vi "getSpeedAndGainSettings.vi"(6 "Delay between send and receive [ms]":i32=100, 8 "error in (no error)":errorcluster, 11 "CCD in":refnum<class "CCD.lvclass">) -> (0 "error out":errorcluster, 1 "CCD-gain options":string[](array[string]), 2 "CCD-speed options":string[](array[string]), 3 "CCD out":refnum<class "CCD.lvclass">)   [LabVIEW 2023, in "CCD.lvclass"]
doc: "Wrapper around the getSpeed and getGain VIs for convenience."
uses:
  CCD.lvclass
  CCD.lvclass/CCD.ctl
  20f7d3bd-08ac-4524-9bed-df36c1da25a0.vi
  GenericDevice/GenericDevice.lvclass
  <vilib>/JDP Science/JSONtext/JSONtext.lvlib
panel:
  out "results-JSON string":string
  # "Connector Pane"
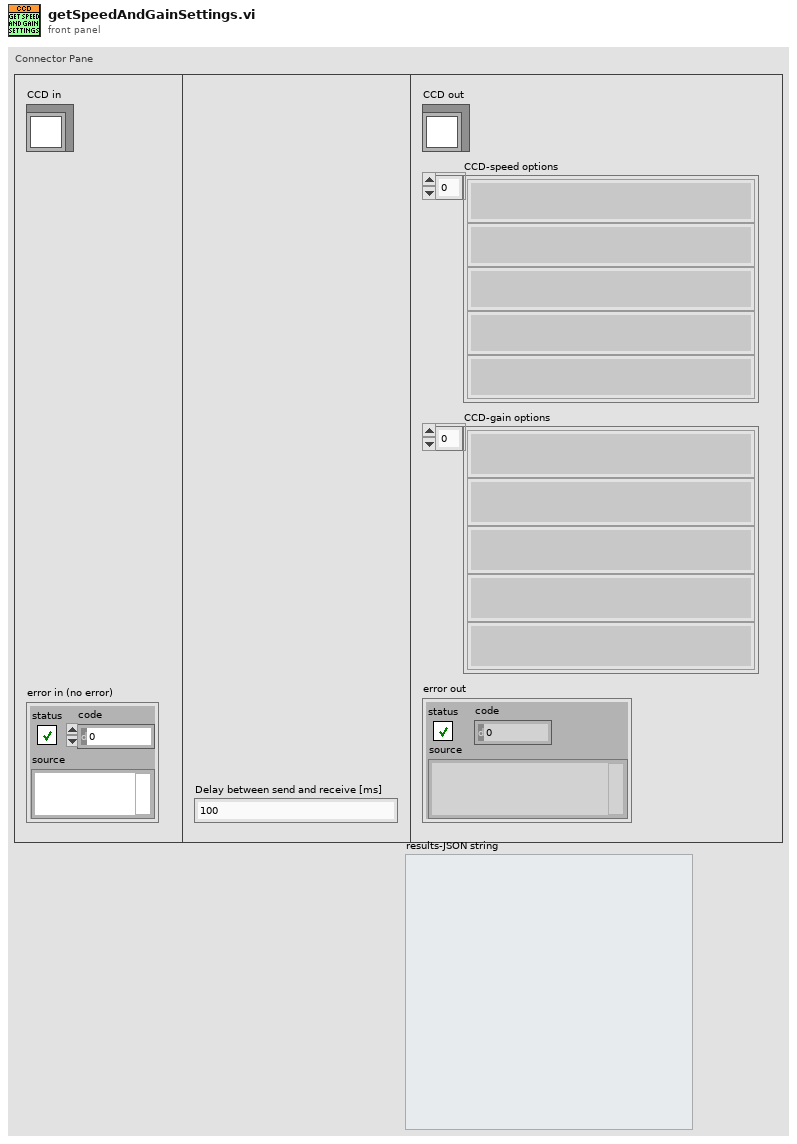
[diagram p1: front panel]
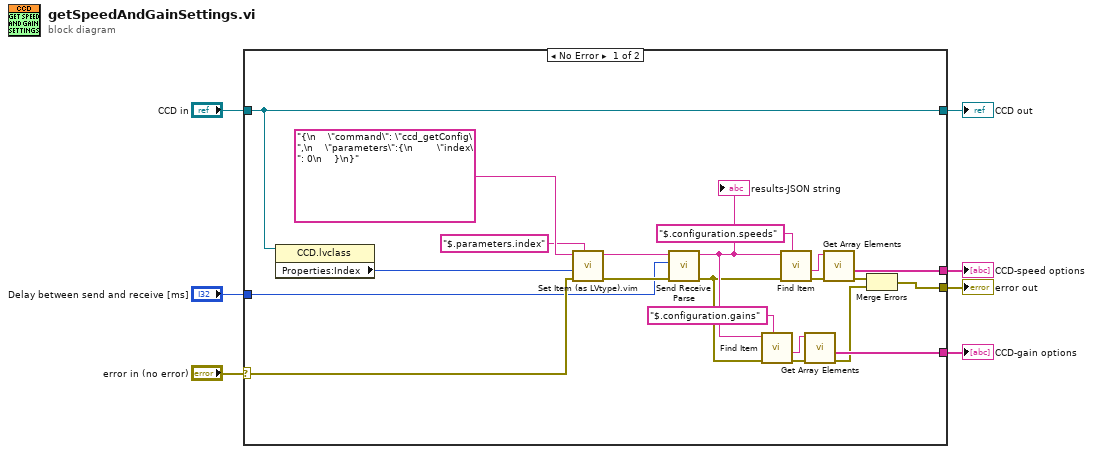
[diagram p0: block diagram]
diagram:
  n1 = case shown="No Error" "error in (no error)" {
    selector: "error in (no error)" -> [w24 w30]
    tunnel: [w20 w30] -> w6
    tunnel: [w26 w29] -> w4
    tunnel: "CCD in" -> [w26 w29]
    tunnel: "Delay between send and receive [ms]" -> [w22 _]
    tunnel: [w16 _] -> w2
    tunnel: [w9 _] -> w1
    frame No Error {
      n2 = property class="CCD.lvclass"(reference=w26) -> ("Properties:Index"=w25:i32)  [unwired: 1 in, 2 out]
      n3 = call "Set Item (as LVtype).vim"("$Path or Item Name"="$.parameters.index", "error in (no error)"=w24, "Anything"=w25, "JSON"="{\n    \"command\": \"ccd_getConfig\",\n    \"parameters\":{\n        \"index\": 0\n    }\n}") -> ("error out"=w23:errorcluster, "<JSON>"=w8:string)  [unwired: 4 in, 1 out]
      n4 = call "Send Receive Parse.vi"("error in"=w23, "Delay between send and receive [ms]"=w22, "<JSON>"=w8) -> ("error out"=w15:errorcluster, "results-JSON string"=w19:string)  [unwired: 6 in, 1 out]
      "results-JSON string" <- w19
      n5 = call <vilib>:"Find Item.vi"("$Path or Item Name"="$.configuration.gains", "error in (no error)"=w15, "JSON"=w19) -> ("error out"=w14:errorcluster, "<JSON>"=w17:string)  [unwired: 5 in, 2 out]
      n6 = call <vilib>:"Find Item.vi"("$Path or Item Name"="$.configuration.speeds", "error in (no error)"=w15, "JSON"=w19) -> ("error out"=w12:errorcluster, "<JSON>"=w11:string)  [unwired: 5 in, 2 out]
      n7 = call <vilib>:"Get Array Elements.vi"("error in (no error)"=w14, "JSON"=w17) -> ("error out"=w13:errorcluster, "<JSON>"=w16:string[])  [unwired: 7 in, 1 out]
      n8 = call <vilib>:"Get Array Elements.vi"("error in (no error)"=w12, "JSON"=w11) -> ("error out"=w10:errorcluster, "<JSON>"=w9:string[])  [unwired: 7 in, 1 out]
      n9 = Merge Errors(w10, w13) -> (w20:errorcluster)
    }
    frame Error {
    }
  }
  "error out" <- w6
  "CCD out" <- w4
  "CCD-gain options" <- w2
  "CCD-speed options" <- w1
